vi "set direct sampling.vi"(8 "error in (no error)":errorcluster, 10 "Direct Sampling State":T1, 11 "DeviceRefnum":u64) -> (0 "error out":errorcluster, 2 "function return":i32, 3 "DeviceRefnum Out":u64)   [LabVIEW 2015, in "rtlsdr.lvlib"]
doc: "Enable or disable the direct sampling mode. When enabled, the IF mode of the RTL2832 is activated, and rtlsdr_set_center_freq() will control the IF-frequency of the DDC, which can be used to tune from 0 to 28.8 MHz (xtal frequency of the RTL2832)."
uses:
  rtlsdr.lvlib
  rtlsdr/rtlsdr.dll
  controls/Direct Sampling States.ctl
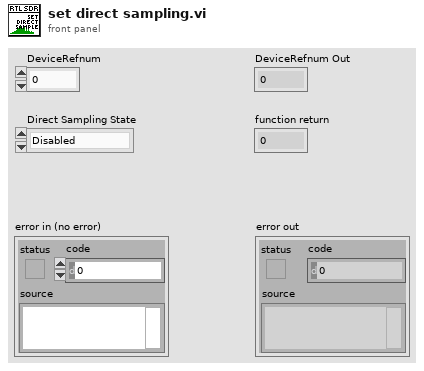
[diagram p1: front panel]
types:
  T1 = typedef "rtlsdr.lvlib/Direct Sampling States.ctl" = enum16{"Disabled", "I-ADC Input Enabled", "Q-ADC Input Enabled"}
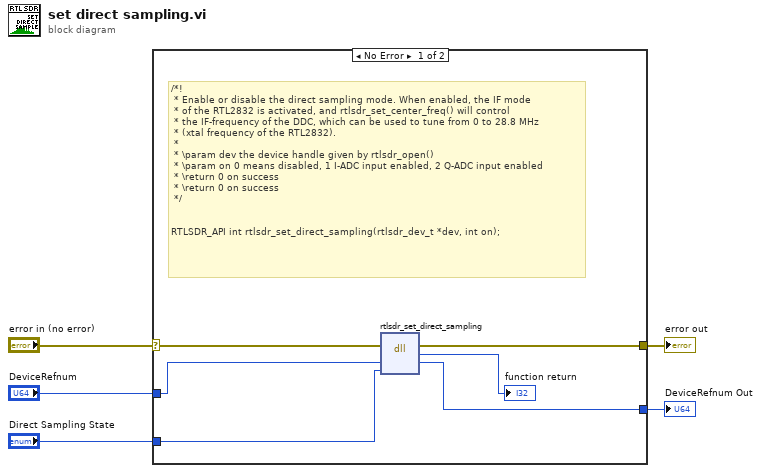
[diagram p0: block diagram]
diagram:
  n1 = case shown="No Error" "error in (no error)" {
    selector: "error in (no error)" -> [w6 w13]
    tunnel: [w10 w13] -> w5
    tunnel: "DeviceRefnum" -> [w9 w12]
    tunnel: [w8 w12] -> w3
    tunnel: "Direct Sampling State" -> [w7 _]
    frame No Error {
      # "/*!\n * Enable or disable the direct sampling mode. When enabled, the IF mode\n * of the RTL2832 is activated, and rtlsdr_set_center_freq() will control\n * the IF-frequency of the DDC, which can be used to tune from 0 to 28.8 MHz\n * (xtal frequency of the RTL2832).\n *\n * \\param dev the device handle given by rtlsdr_open()\n * \\param on 0 means disabled, 1 I-ADC input enabled, 2 Q-ADC input enabled\n * \\return 0 on success\n * \\return 0 on success\n */\n\n\nRTLSDR_API int rtlsdr_set_direct_sampling(rtlsdr_dev_t *dev, int on);"
      n2 = dll-call lib="C:/Users/TheDoctor/Documents/Projects/Labview Libraries/rtlsdr/rtlsdr.*" fn="rtlsdr_set_direct_sampling"(error in=w6, "DeviceRefnum"=w9, "Direct Sampling State"=w7) -> (error out=w10:errorcluster, "return type"=→"function return":i32, "DeviceRefnum"=w8:u64)  [unwired: 3 in, 1 out]
    }
    frame Error {
    }
  }
  "error out" <- w5
  "DeviceRefnum Out" <- w3
